vi "数值变换.vi"(3 "error in (no error)":errorcluster caption="错误输入（无错误）", 4 "比例":dbl=10000.0 format="%#_13g", 5 "数值":dbl) -> (0 "error out":errorcluster caption="错误输出", 2 "数值变换输出":u32[](array[numeric]))   [LabVIEW 2015, in "MSP6715.lvlib"]
uses:
  MSP6715.lvlib
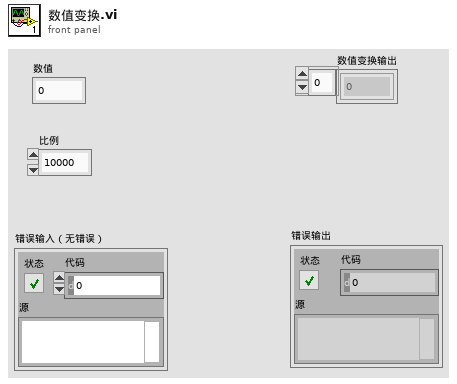
[diagram p1: front panel]
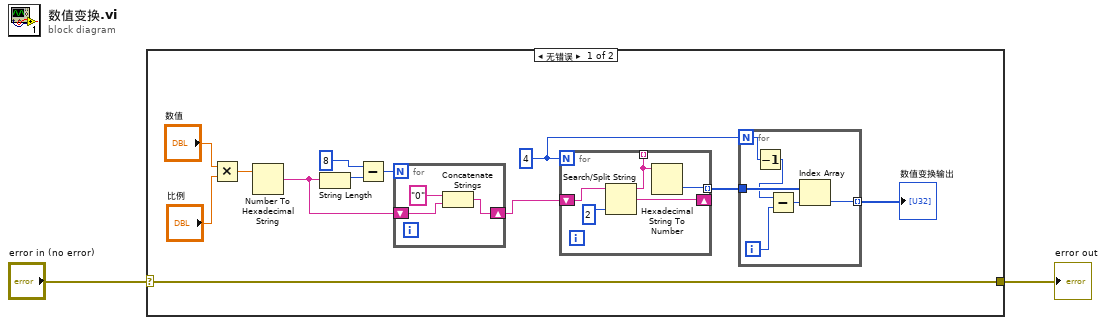
[diagram p0: block diagram]
diagram:
  n1 = case shown="无错误" "error in (no error)" {
    selector: "error in (no error)" -> [w3 w29]
    tunnel: [w3 w29] -> w1
    frame No Error {
      w5 = 4
      n2 = Multiply(x="数值", y="比例") -> (x*y=w12:dbl)
      n3 = Number To Hexadecimal String(2:w12) -> (0:w8:string)  [unwired: 1 in]
      n4 = String Length(string=w8) -> (length=w10:i32)
      n5 = Subtract(x=8, y=w10) -> (x-y=w9:i32)
      n6 = for {
        N: w9 -> [_]
        shift-right: [w26] -> w7
        shift-left: w8 -> [w28]
        n7 = Concatenate Strings("0", w28) -> (w26:string)
      }
      n8 = for {
        N: w5 -> [_]
        shift-right: [w23] -> _
        shift-left: w7 -> [w25]
        tunnel: [w22] -> w6 mode=indexing
        tunnel: [w21] -> _ mode=indexing
        n9 = Search/Split String(string=w25, offset (0)=2 ("长度（剩余）")) -> (substring before match=w21:string, match + rest of string=w23:string)  [unwired: 1 in, 1 out]
        n10 = Hexadecimal String To Number(string=w21) -> (number=w22:u32)  [unwired: 2 in, 1 out]
      }
      n11 = for {
        N: w5 -> [w16]
        tunnel: w6 -> [w20]
        tunnel: [w17] -> w4 mode=indexing
        i -> [w18]
        n12 = Decrement(x=w16) -> (x-1=w15:i32)
        n13 = Subtract(x=w15, y=w18) -> (x-y=w19:i32)
        n14 = Index Array(array=w20, index=w19) -> (element=w17:u32)
      }
      "数值变换输出" <- w4
    }
    frame Error {
    }
  }
  "error out" <- w1
